vi "cost func.vi"(2 "Y":dbl[][](array[numeric]), 3 "AL":dbl[][](array[numeric])) -> (0 "loss":dbl, 1 "Accuracy":dbl)   [LabVIEW 2020]
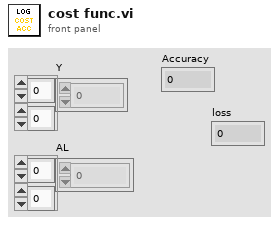
[diagram p1: front panel]
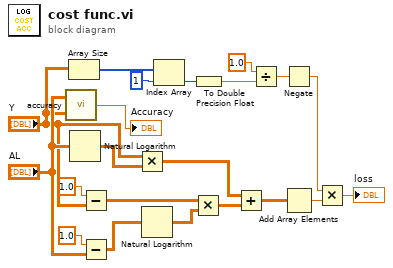
[diagram p0: block diagram]
diagram:
  n1 = call "accuracy.vi"("Y_actual"="Y", "Y_predicted"="AL") -> ("Accuracy"=→"Accuracy":dbl)
  n2 = Array Size(array="Y") -> (size(s)=w7:i32[])
  n3 = Natural Logarithm(1:"AL") -> (0:w21:dbl[][])
  n4 = Subtract(x=1.0, y="Y") -> (x-y=w16:dbl[][])
  n5 = Subtract(x=1.0, y="AL") -> (x-y=w18:dbl[][])
  n6 = Multiply(x="Y", y=w21) -> (x*y=w15:dbl[][])
  n7 = Natural Logarithm(1:w18) -> (0:w17:dbl[][])
  n8 = Index Array(array=w7, index=1) -> (element=w4:i32)
  n9 = Multiply(x=w16, y=w17) -> (x*y=w14:dbl[][])
  n10 = To Double Precision Float(number=w4) -> (double precision float=w5:dbl)
  n11 = Add(x=w15, y=w14) -> (x+y=w13:dbl[][])
  n12 = Divide(x=1.0, y=w5) -> (x/y=w11:dbl)
  n13 = Negate(x=w11) -> (-x=w10:dbl)
  n14 = Add Array Elements(numeric array=w13) -> (sum=w9:dbl)
  n15 = Multiply(x=w10, y=w9) -> (x*y=→"loss":dbl)
